vi "KVP to Tree.vi"(9 "KVP":variant, 11 "Root Node":variant) -> (3 "Variant Tree":variant)   [LabVIEW 2013, in "OpenVariant.lvlib"]
uses:
  OpenVariant.lvlib
  Conversions/OpenConvert.lvlib
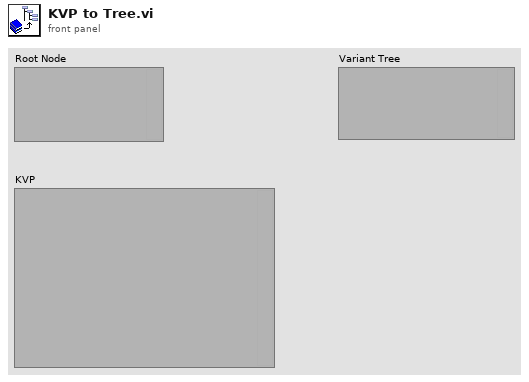
[diagram p1: front panel]
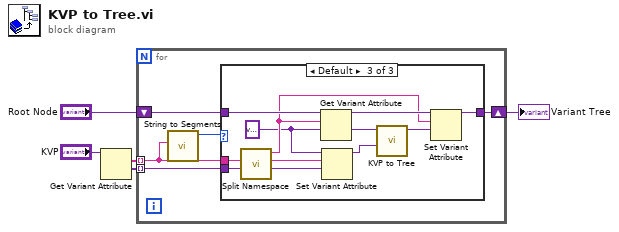
[diagram p0: block diagram]
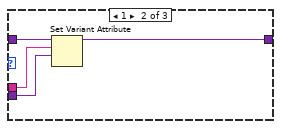
[diagram p3: hidden frame]
diagram:
  n1 = Get Variant Attribute(Variant="KVP") -> (names=w4:string[], values=w5:variant[])  [unwired: 3 in, 2 out]
  n2 = for {
    tunnel: w5 -> [w7] mode=indexing
    tunnel: w4 -> [w6] mode=indexing
    shift-right: [w9] -> w3
    shift-left: "Root Node" -> [w10]
    n3 = call "String to Segments.vi"("String"=w6) -> ("Nb segments"=w8:i32)  [unwired: 9 in, 1 out]
    n4 = case shown="Default" w8 {
      tunnel: w10 -> [w11 w15 w25]
      tunnel: [w11 w12 w18] -> w9
      tunnel: w6 -> [_ w14 w26]
      tunnel: w7 -> [_ w13 w22]
      frame 0 {
      }
      frame 1 {
        n5 = Set Variant Attribute(Variant=w15, name=w14, value=w13) -> (Variant out=w12:variant)  [unwired: 1 in, 2 out]
      }
      frame Default {
        w16 = variant ("default value (empty variant)")
        n6 = call "Split Namespace.vi"("Namespaced String"=w26) -> ("String"=w23:string, "Namespace"=w17:string)  [unwired: 9 in]
        n7 = Get Variant Attribute(Variant=w25, name=w17, default value (empty Variant)=w16) -> (duplicate Variant=w24:variant, value=w20:variant)  [unwired: 1 in, 2 out]
        n8 = Set Variant Attribute(Variant=w16, name=w23, value=w22) -> (Variant out=w19:variant)  [unwired: 1 in, 2 out]
        n9 = call "KVP to Tree.vi"("KVP"=w19, "Root Node"=w20) -> ("Variant Tree"=w21:variant)  [unwired: 9 in]
        n10 = Set Variant Attribute(Variant=w24, name=w17, value=w21) -> (Variant out=w18:variant)  [unwired: 1 in, 2 out]
      }
    }
  }
  "Variant Tree" <- w3
